vi "validate.vi"(8 "error in":errorcluster, 11 "Polynomial Scale configuration in":refnum<class "Polynomial Scale configuration.lvclass">) -> (0 "error out":errorcluster, 3 "Polynomial Scale configuration out":refnum<class "Polynomial Scale configuration.lvclass">)   [LabVIEW 2013, in "Polynomial Scale configuration.lvclass"]
doc: "This function performs validation of the configuration. This function should be safe to call at any point and should not rely on anything in the runtime environment."
uses:
  Polynomial Scale configuration.lvclass
  <vilib>/NI/DCAF Templates/DCAF Scaling/module/configuration/Scaling configuration.lvclass
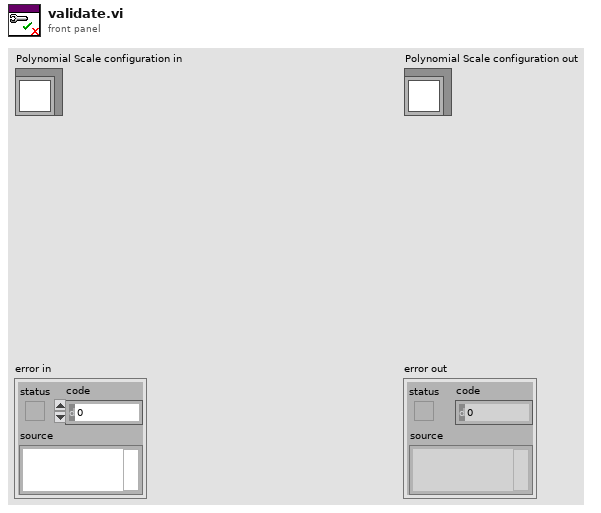
[diagram p1: front panel]
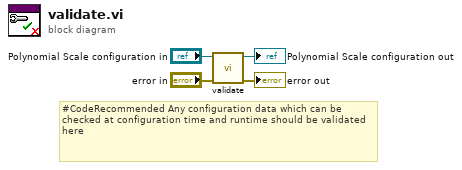
[diagram p0: block diagram]
diagram:
  # "#CodeRecommended Any configuration data which can be checked at configuration time and runtime should be validated here"
  n1 = call-parent "validate.vi"("error in"="error in", "Scaling configuration in"="Polynomial Scale configuration in") -> ("error out"=→"error out":errorcluster, "Scaling configuration out"=→"Polynomial Scale configuration out":refnum<class "Polynomial Scale configuration.lvclass">)  [unwired: 8 in]
